vi "Stop Core.vi"(10 "final error code":i32, 11 "IMAQdx Cam Actor in":refnum<class "IMAQdx Cam Actor.lvclass">) -> (3 "IMAQdx Cam Actor out":refnum<class "IMAQdx Cam Actor.lvclass">)   [LabVIEW 2014, in "IMAQdx Cam Actor.lvlib" / "IMAQdx Cam Actor.lvclass"]
doc: "(<B>Filename</B>: Actor Framework.lvlib:Actor.lvclass:Stop Core.vi)\n\nDefines what the actor does before it stops. Use the <B>final error code</B> input to determine whether the actor shut down in response to an error.\n\nBy default, this method does nothing. A descendant class may override it to define behavior, such as shutting down any processes the actor initiated in its override of the Actor Core method."
uses:
  IMAQdx Cam Actor.lvclass
  <vilib>/ActorFramework/Actor/Actor.lvclass
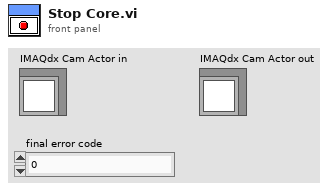
[diagram p1: front panel]
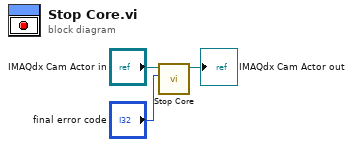
[diagram p0: block diagram]
diagram:
  n1 = call-parent "Stop Core.vi"("final error code"="final error code", "Actor in"="IMAQdx Cam Actor in") -> ("Actor out"=→"IMAQdx Cam Actor out":refnum<class "IMAQdx Cam Actor.lvclass">)  [unwired: 9 in]
